vi "preprocessing.vi"() -> ()   [LabVIEW 2025]
uses:
  <vilib>/numeric/Random Number (Range) DBL.vi
panel:
  out "Table 5":string[][](table)
  out "potencia ativa 3":dbl[](graph) caption="potencia ativa"
  out "Table 4":string[][](table)
  out "Table":string[][](table)
  out "potencia ativa 2":dbl[](graph) caption="potencia ativa"
  out "Table 3":string[][](table)
  in  "limite inferior 0,80":dbl
  in  "limite superior 0,95":dbl=100.0
  out "potencia ativa":dbl[](graph)
  out "Table 2":string[][](table)
  out "tensao A":string[][](table)
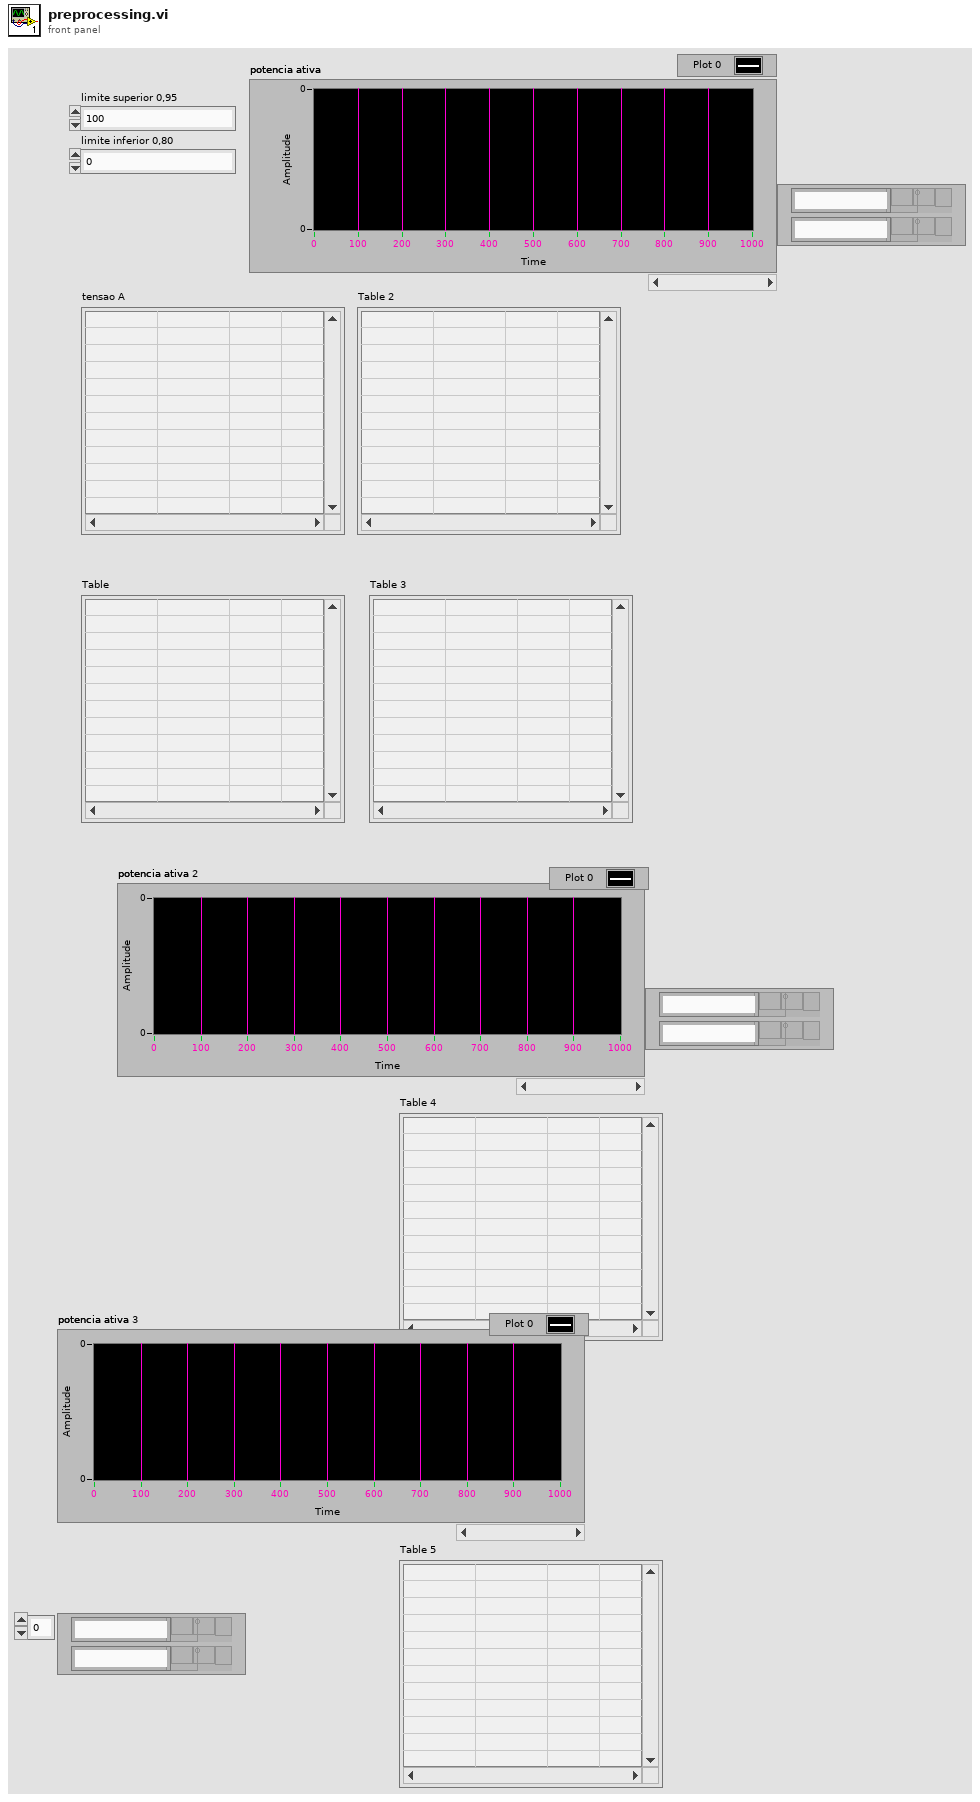
[diagram p1: front panel]
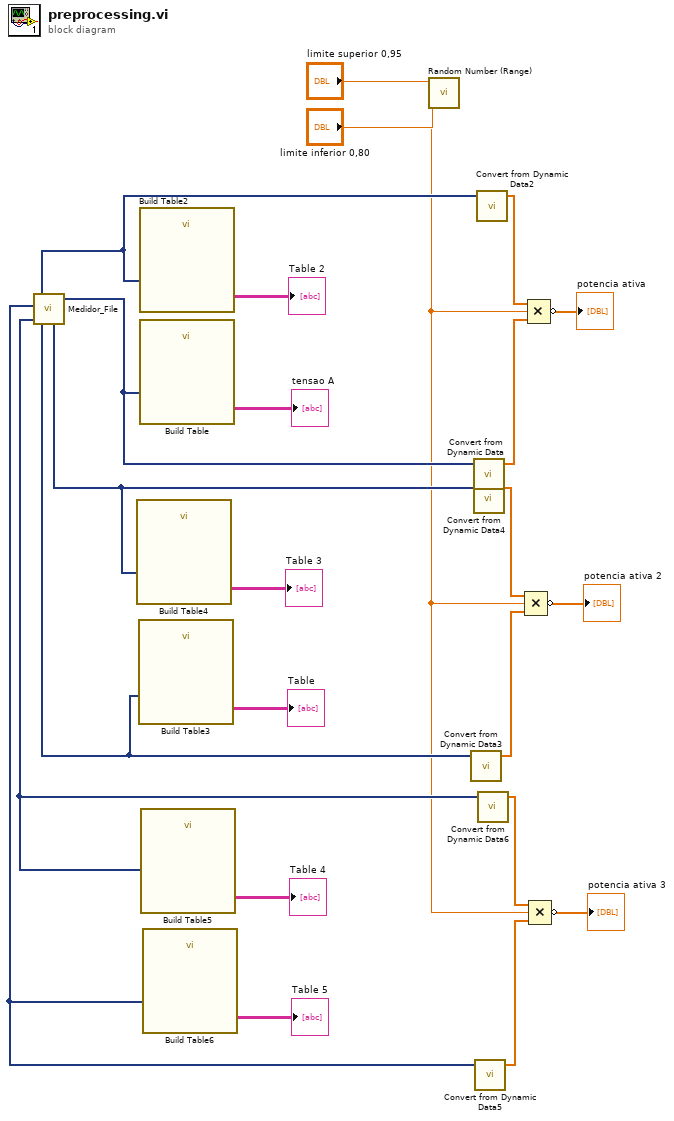
[diagram p0: block diagram]
diagram:
  n1 = call "Medidor_File.vi"() -> ("Corrente Fase C"=w3:dynamicdata, "Corrente Fase B"=w11:dynamicdata, "Corrente Fase A"=w21:dynamicdata, "Tensão Fase C"=w10:dynamicdata, "Tensão Fase B"=w2:dynamicdata, "Tensão Fase A"=w19:dynamicdata)  [unwired: 1 out]
  n2 = call "Build Table4"("Signals"=w11) -> ("Table"=→"Table 3":string[][])  [unwired: 4 in, 6 out]
  n3 = call "Build Table3"("Signals"=w10) -> ("Table"=→"Table":string[][])  [unwired: 4 in, 6 out]
  n4 = call "Build Table2"("Signals"=w19) -> ("Table"=→"Table 2":string[][])  [unwired: 4 in, 6 out]
  n5 = call "Build Table"("Signals"=w21) -> ("Table"=→"tensao A":string[][])  [unwired: 4 in, 6 out]
  n6 = call "Build Table5"("Signals"=w3) -> ("Table"=→"Table 4":string[][])  [unwired: 4 in, 6 out]
  n7 = call "Build Table6"("Signals"=w2) -> ("Table"=→"Table 5":string[][])  [unwired: 4 in, 6 out]
  n8 = call-poly <vilib>:"Random Number (Range).vi"("lower bound (0)"="limite inferior 0,80", "upper bound (100)"="limite superior 0,95") -> ("number"=w1:dbl)  [unwired: 9 in]
  n9 = call "Convert from Dynamic Data3"("Dynamic Data Type"=w10) -> ("Array"=w14:dbl[])  [unwired: 3 in]
  n10 = call "Convert from Dynamic Data"("Dynamic Data Type"=w21) -> ("Array"=w23:dbl[])  [unwired: 3 in]
  n11 = call "Convert from Dynamic Data4"("Dynamic Data Type"=w11) -> ("Array"=w15:dbl[])  [unwired: 3 in]
  n12 = call "Convert from Dynamic Data5"("Dynamic Data Type"=w2) -> ("Array"=w7:dbl[])  [unwired: 3 in]
  n13 = call "Convert from Dynamic Data2"("Dynamic Data Type"=w19) -> ("Array"=w24:dbl[])  [unwired: 3 in]
  n14 = call "Convert from Dynamic Data6"("Dynamic Data Type"=w3) -> ("Array"=w8:dbl[])  [unwired: 3 in]
  n15 = Compound Arithmetic op=MULTIPLY(w15, w1, w14) -> (invert →"potencia ativa 2":dbl[])
  n16 = Compound Arithmetic op=MULTIPLY(w24, w1, w23) -> (invert →"potencia ativa":dbl[])
  n17 = Compound Arithmetic op=MULTIPLY(w8, w1, w7) -> (invert →"potencia ativa 3":dbl[])
